vi "format display.vi"(6 "Channel":dbl(slide)=1.0 min=0.0 max=7.0 step=1.0 scale=0.0..7.0, 8 "Gain":dbl[](array[numeric])=[1.0, 1.0, 1.0, 1.0, 1.0, 1.0, 1.0, 1.0], 9 "Display":enum16{"X and Y", "R and Theta"}(ring), 10 "Results (X,Y,R,Theta)":dbl[][](array[numeric]), 11 "t0":timestamp) -> (0 "X/R":dbl, 1 "Array 2":cluster{dbl[], dbl[]}[](array[cluster]), 2 "Y/Theta Array":waveform(dbl)[](array[waveform]), 3 "X/R Array":waveform(dbl)[](array[waveform]), 4 "Y/R":dbl)   [LabVIEW 2013]
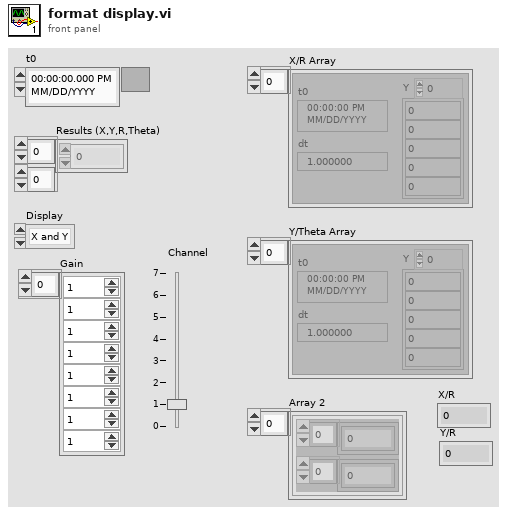
[diagram p1: front panel]
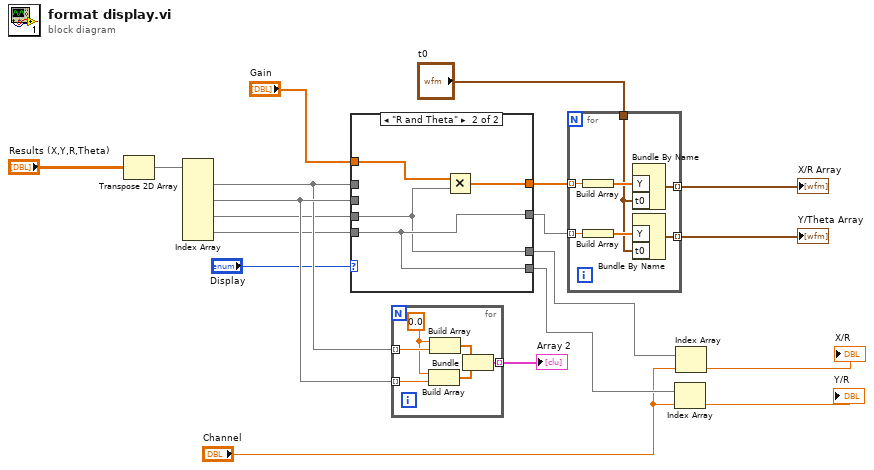
[diagram p0: block diagram]
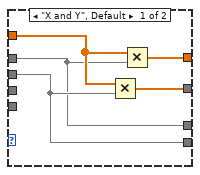
[diagram p2: hidden frame]
diagram:
  n1 = Transpose 2D Array(2D array="Results (X,Y,R,Theta)") -> (transposed array=w9:dbl[][])
  n2 = Index Array(array=w9) -> (element #1=w16:dbl[], element #2=w17:dbl[], element #3=w12:dbl[], element #4=w13:dbl[])  [unwired: 8 in]
  n3 = case shown="\"R and Theta\"" "Display" {
    tunnel: w16 -> [w20 _]
    tunnel: [w23 w27] -> w7
    tunnel: w17 -> [w21 _]
    tunnel: [w22 w26] -> w6
    tunnel: w12 -> [_ w25]
    tunnel: w13 -> [_ w26]
    tunnel: "Gain" -> [w24 w28]
    tunnel: [w21 w26] -> w2
    tunnel: [w20 w25] -> w3
    frame "X and Y", Default {
      n4 = Multiply(x=w24, y=w21) -> (x*y=w22:dbl[])
      n5 = Multiply(x=w24, y=w20) -> (x*y=w23:dbl[])
    }
    frame "R and Theta" {
      n6 = Multiply(x=w28, y=w25) -> (x*y=w27:dbl[])
    }
  }
  n7 = for {
    tunnel: w16 -> [w34] mode=indexing
    tunnel: w17 -> [w33] mode=indexing
    tunnel: [w29] -> w18 mode=indexing
    w32 = 0.0
    n8 = Build Array(w32, w33) -> (w30:dbl[])
    n9 = Build Array(w32, w34) -> (w31:dbl[])
    n10 = Bundle(w31, w30) -> (w29:cluster{dbl[], dbl[]})  [unwired: 1 in]
  }
  "Array 2" <- w18
  n11 = for {
    tunnel: w7 -> [w41] mode=indexing
    tunnel: w6 -> [w40] mode=indexing
    tunnel: [w39] -> w15 mode=indexing
    tunnel: [w38] -> w19 mode=indexing
    tunnel: "t0" -> [w35]
    n12 = Build Array(w41) -> (w37:dbl[])
    n13 = Build Array(w40) -> (w36:dbl[])
    n14 = Bundle By Name("Y"=w37, "t0"=w35) -> (w39:waveform(dbl))  [unwired: 1 in]
    n15 = Bundle By Name("Y"=w36, "t0"=w35) -> (w38:waveform(dbl))  [unwired: 1 in]
  }
  "Y/Theta Array" <- w19
  "X/R Array" <- w15
  n16 = Index Array(array=w2, index="Channel") -> (element=→"Y/R":dbl)
  n17 = Index Array(array=w3, index="Channel") -> (element=→"X/R":dbl)
